vi "Place dots fixed.vi"(6 "Right Corner":cluster{"X":sgl, "Y":sgl}[](array[cluster]), 8 "Left Height":dbl, 9 "Left Orientation":dbl, 10 "Left Corner":cluster{"X":sgl, "Y":sgl}[](array[cluster]), 11 "Image IN":T1) -> (3 "Image OUT":T1)   [LabVIEW 2018]
uses:
  <vilib>/vision/Image Controls.llb/IMAQ Image.ctl
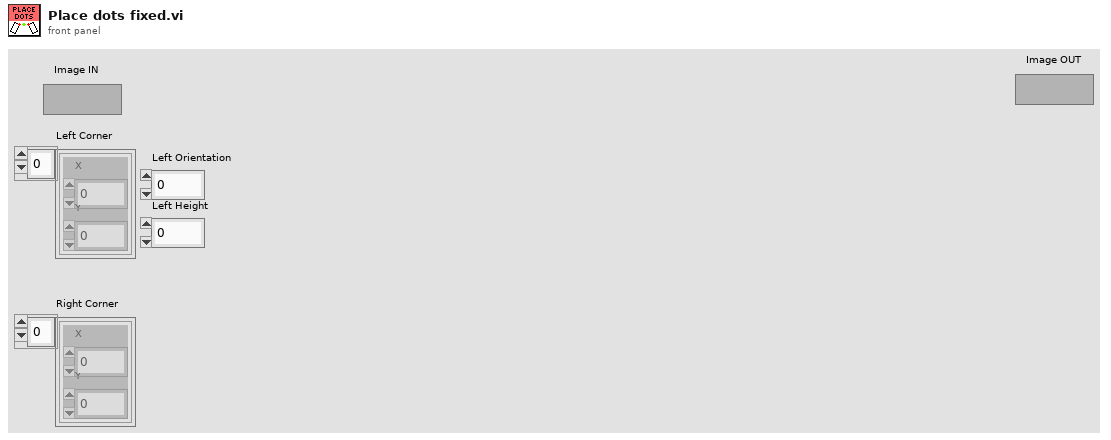
[diagram p1: front panel]
types:
  T1 = typedef "IMAQ Image.ctl" = refnum<image>
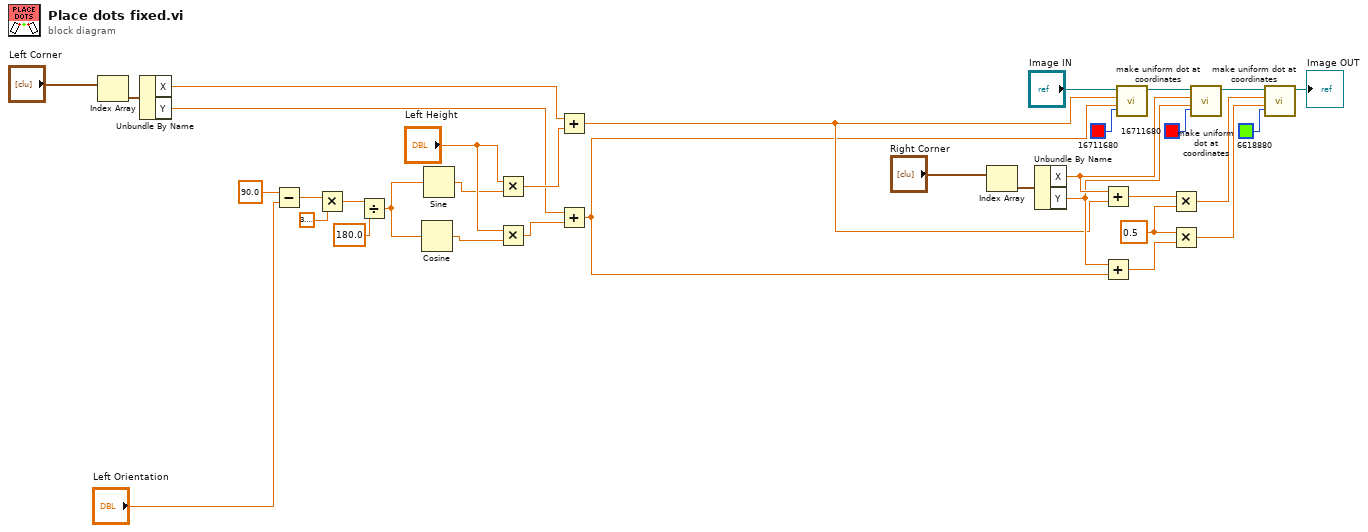
[diagram p0: block diagram]
diagram:
  w13 = 0.5 ("x")
  n1 = Index Array(array="Left Corner") -> (element=w33:cluster{"X":sgl, "Y":sgl})  [unwired: 1 in]
  n2 = Unbundle By Name(w33) -> ("X"=w19:sgl, "Y"=w18:sgl)
  n3 = Subtract(x=90.0, y="Left Orientation") -> (x-y=w29:dbl)
  n4 = Multiply(x=w29, y=3.141592653589793) -> (x*y=w27:dbl)
  n5 = Divide(x=w27, y=180.0) -> (x/y=w25:dbl)
  n6 = Cosine(x=w25) -> (cos(x)=w22:dbl)
  n7 = Sine(x=w25) -> (sin(x)=w23:dbl)
  n8 = Multiply(x="Left Height", y=w23) -> (x*y=w21:dbl)
  n9 = Multiply(x="Left Height", y=w22) -> (x*y=w20:dbl)
  n10 = Add(x=w19, y=w21) -> (x+y=w10:dbl)
  n11 = Add(x=w18, y=w20) -> (x+y=w9:dbl)
  n12 = Index Array(array="Right Corner") -> (element=w32:cluster{"X":sgl, "Y":sgl})  [unwired: 1 in]
  n13 = Unbundle By Name(w32) -> ("X"=w16:sgl, "Y"=w15:sgl)
  n14 = Add(x=w16, y=w10) -> (x+y=w14:dbl)
  n15 = Add(x=w15, y=w9) -> (x+y=w12:dbl)
  n16 = call "make uniform dot at coordinates.vi"("Color"=u32 16711680, "Y"=w9, "X"=w10, "Refnum in"="Image IN") -> ("Refnum out"=w8:T1)  [unwired: 7 in]
  n17 = Multiply(x=w14, y=w13) -> (x*y=w5:dbl)
  n18 = Multiply(x=w13, y=w12) -> (x*y=w4:dbl)
  n19 = call "make uniform dot at coordinates.vi"("Color"=u32 16711680, "Y"=w15, "X"=w16, "Refnum in"=w8) -> ("Refnum out"=w6:T1)  [unwired: 7 in]
  n20 = call "make uniform dot at coordinates.vi"("Color"=u32 6618880, "Y"=w4, "X"=w5, "Refnum in"=w6) -> ("Refnum out"=→"Image OUT":T1)  [unwired: 7 in]
